vi "Arcade Drive Implementation.vi"(10 "Right Setpoint":dbl, 11 "Left Setpoint":dbl) -> (2 "Numeric":dbl, 3 "Numeric 2":dbl)   [LabVIEW 2019]
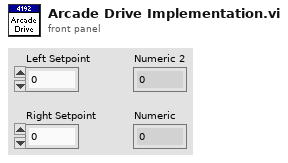
[diagram p1: front panel]
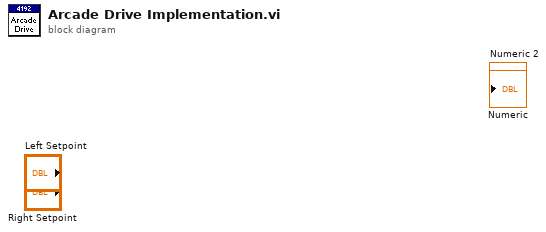
[diagram p0: block diagram]
diagram:
